vi "testError.vi"() -> (0 "error out":errorcluster)   [LabVIEW 2019, in "AssertionTest.lvlib" / "AssertStringContainsString.lvlib"]
uses:
  AssertStringContainsString.lvlib
  <vilib>/Utility/error.llb/Error Cluster From Error Code.vi
  <vilib>/ErrorRing/Error Ring.xnode
  Assertion/Assertion.lvlib
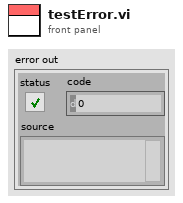
[diagram p1: front panel]
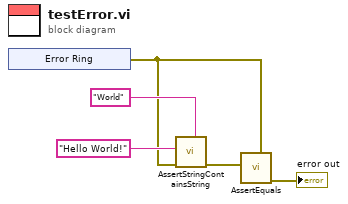
[diagram p0: block diagram]
diagram:
  n1 = xnode "Error Ring"() -> ("error out"=w2:errorcluster)
  n2 = call "AssertStringContainsString.vi"("Needle"="World", "error in (no error)"=w2, "Haystack"="Hello World!") -> ("error out"=w3:errorcluster)  [unwired: 7 in, 1 out]
  n3 = call "AssertEquals.vi"("Expected"=w2, "Actual"=w3) -> ("error out"=→"error out":errorcluster)  [unwired: 8 in, 1 out]
